vi "CAL_GCP_R_fpga.vi"(11 "R_ROLL":sgl) -> (0 "R_Period":i16, 1 "R_GCP":sgl, 3 "R_NUM":u32)   [LabVIEW 2019]
panel:
  in  "IMU_init_R":sgl
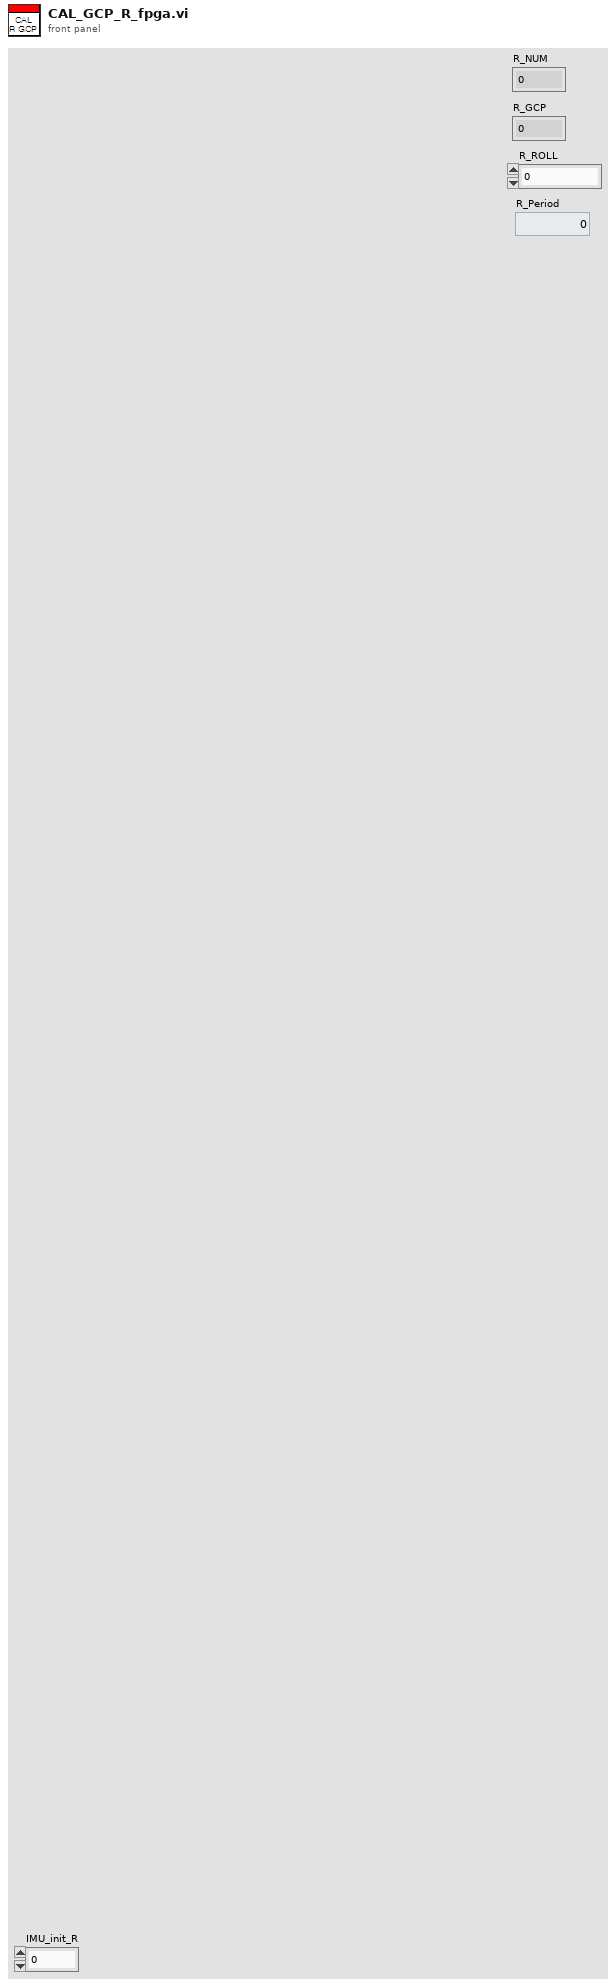
[diagram p1: front panel]
types:
  T1 = enum16{"Init", "HF", "Cross", "HE", "Cross_E", "Init_F"}
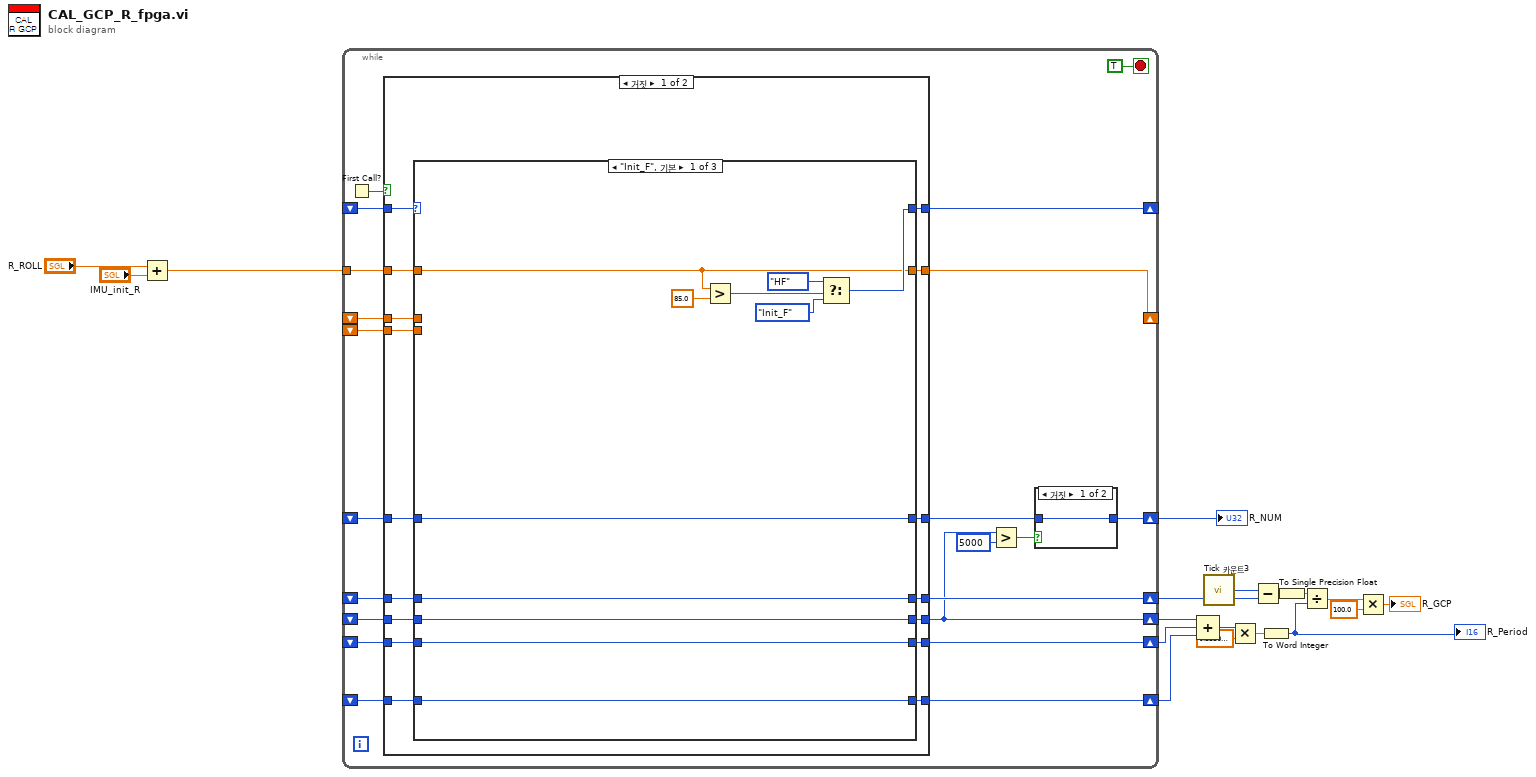
[diagram p0: block diagram]
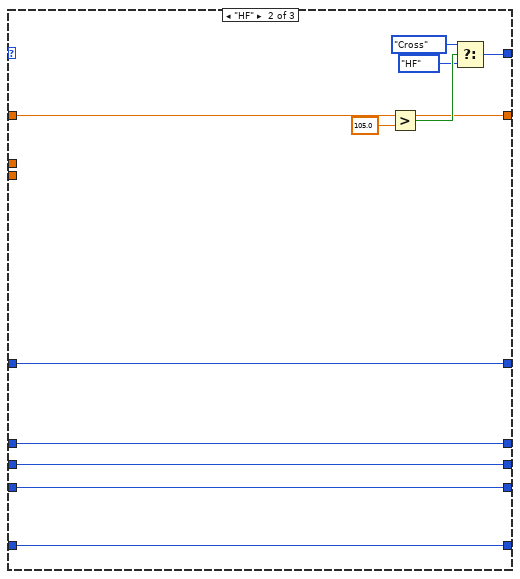
[diagram p2: hidden frame]
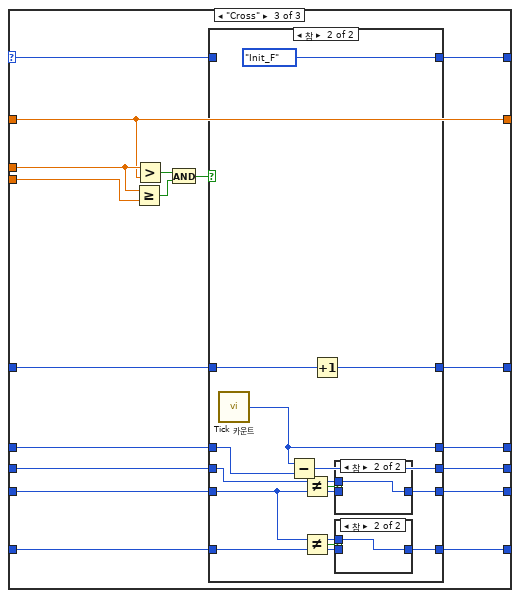
[diagram p3: hidden frame]
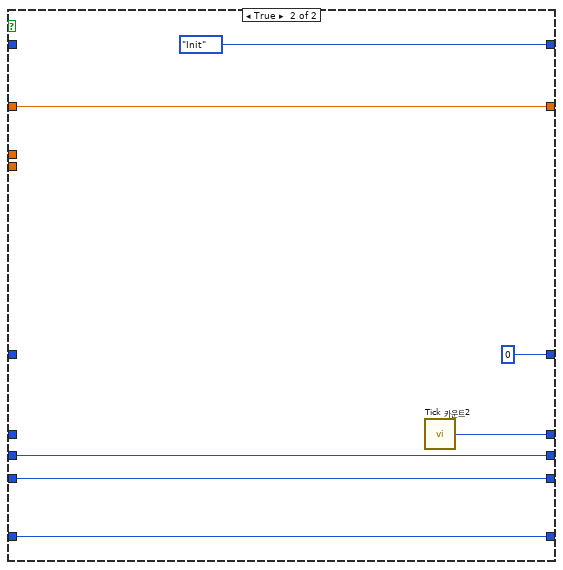
[diagram p7: hidden frame]
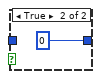
[diagram p8: hidden frame]
diagram:
  n1 = Add(x="R_ROLL", y="IMU_init_R") -> (x+y=w10:sgl)
  n2 = while {
    tunnel: w10 -> [w36]
    shift-right: [w21] -> _
    shift-left: _ -> [w20]
    shift-right: [w37] -> _
    shift-left: _ -> [w34]
    shift-left: _ -> [w33]
    shift-right: [w30] -> w13
    shift-left: _ -> [w35]
    shift-right: [w26] -> w6
    shift-left: _ -> [w25]
    shift-right: [w23] -> w5
    shift-left: _ -> [w24]
    shift-right: [w28] -> w12
    shift-left: _ -> [w27]
    shift-right: [w19] -> w7
    shift-left: _ -> [w22]
    stop <- TRUE stop-if-true
    n3 = First Call?() -> (First Call?: T/F=w38:bool)
    n4 = case shown="거짓" w38 {
      tunnel: [w54 w125] -> w37
      tunnel: w36 -> [w55 w125]
      tunnel: w35 -> [w52 _]
      tunnel: [w53 u32 0] -> w29
      tunnel: w34 -> [w51 _]
      tunnel: w33 -> [w50 _]
      tunnel: [w49 w119] -> w28
      tunnel: w27 -> [w48 _]
      tunnel: [w47 w123] -> w26
      tunnel: w25 -> [w46 w123]
      tunnel: w24 -> [w45 w122]
      tunnel: [w44 w122] -> w23
      tunnel: [w43 w121] -> w19
      tunnel: w22 -> [w42 w121]
      tunnel: [w40 T1."Init"] -> w21
      tunnel: w20 -> [w41 _]
      frame False {
        n5 = case shown="\"Init_F\", 기본" w41 {
          selector: w41 -> [_ _ w95]
          tunnel: w55 -> [w63 w76 w88]
          tunnel: [w63 w76 w88] -> w54
          tunnel: [w62 w75 w90] -> w53
          tunnel: w52 -> [w62 w75 w91]
          tunnel: w51 -> [_ _ w89]
          tunnel: w50 -> [_ _ w94]
          tunnel: [w61 w74 w86] -> w49
          tunnel: w48 -> [w61 w74 w85]
          tunnel: [w59 w73 w84] -> w47
          tunnel: w46 -> [w59 w73 w83]
          tunnel: w45 -> [w58 w72 w82]
          tunnel: [w58 w72 w81] -> w44
          tunnel: [w60 w71 w80] -> w43
          tunnel: w42 -> [w60 w71 w79]
          tunnel: [w64 w68 w78] -> w40
          frame "Init_F", Default {
            n6 = Greater?(x=w63, y=sgl 85.0) -> (0:w57:bool)
            n7 = Select(t=T1."HF", s=w57, f=T1."Init_F") -> (s? t:f=w64:T1)
          }
          frame "HF" {
            n8 = Greater?(x=w76, y=sgl 105.0) -> (0:w77:bool)
            n9 = Select(t=T1."Cross", s=w77, f=T1."HF") -> (s? t:f=w68:T1)
          }
          frame "Cross" {
            n10 = Greater Or Equal?(x=w89, y=w94) -> (x >= y?=w93:bool)
            n11 = Greater?(x=w89, y=w88) -> (0:w87:bool)
            n12 = And(x=w87, y=w93) -> (x .and. y?=w92:bool)
            n13 = case shown="참" w92 {
              tunnel: w95 -> [w100 _]
              tunnel: [w100 T1."Init_F"] -> w78
              tunnel: w91 -> [w101 w106]
              tunnel: [w101 w105] -> w90
              tunnel: [w99 w102] -> w86
              tunnel: w85 -> [w99 w112]
              tunnel: [w98 w111] -> w84
              tunnel: w83 -> [w98 w103]
              tunnel: w82 -> [w97 w110]
              tunnel: [w97 w109] -> w81
              tunnel: [w96 w108] -> w80
              tunnel: w79 -> [w96 w104]
              frame False {
              }
              frame True {
                n14 = call "Tick 카운트"() -> ("Tick Count(mSec)"=w102:u32)
                n15 = Subtract(x=w102, y=w112) -> (x-y=w108:u32)
                n16 = Not Equal?(x=w104, y=w103) -> (x != y?=w114:bool)
                n17 = Not Equal?(x=w103, y=w110) -> (x != y?=w113:bool)
                n18 = Increment(x=w106) -> (x+1=w105:u32)
                n19 = case shown="참" w114 {
                  tunnel: w104 -> [_ w118]
                  tunnel: [w117 w118] -> w111
                  tunnel: w103 -> [w117 _]
                  frame False {
                  }
                  frame True {
                  }
                }
                n20 = case shown="참" w113 {
                  tunnel: w103 -> [_ w116]
                  tunnel: w110 -> [w115 _]
                  tunnel: [w115 w116] -> w109
                  frame False {
                  }
                  frame True {
                  }
                }
              }
            }
          }
        }
      }
      frame True {
        n21 = call "Tick 카운트2"() -> ("Tick Count(mSec)"=w119:u32)
      }
    }
    n22 = Greater?(x=w19, y=u32 5000) -> (0:w31:bool)
    n23 = case shown="거짓" w31 {
      tunnel: [w126 u32 0] -> w30
      tunnel: w29 -> [w126 _]
      frame False {
      }
      frame True {
      }
    }
  }
  "R_NUM" <- w13
  n24 = Compound Arithmetic op=ADD(w7, w6, w5) -> (w4:u32)
  n25 = call "Tick 카운트3"() -> ("Tick Count(mSec)"=w9:u32)
  n26 = Multiply(x=w4, y=sgl 0.333) -> (x*y=w2:sgl)
  n27 = Subtract(x=w9, y=w12) -> (x-y=w16:u32)
  n28 = To Word Integer(number=w2) -> (16bit integer=w1:i16)
  "R_Period" <- w1
  n29 = To Single Precision Float(number=w16) -> (single precision float=w14:sgl)
  n30 = Divide(x=w14, y=w1) -> (x/y=w18:sgl)
  n31 = Multiply(x=w18, y=sgl 100.0) -> (x*y=→"R_GCP":sgl)
